vi "write TBM configuration.vi"(8 "error in":errorcluster, 10 "configuration":refnum<class "TBM configuration.lvclass">, 11 "tag bus configurable plugin editor node in":refnum<class "tag bus configurable plugin editor node.lvclass">) -> (0 "error out":errorcluster, 3 "tag bus configurable plugin editor node out":refnum<class "tag bus configurable plugin editor node.lvclass">)   [LabVIEW 2013, in "tag bus configurable plugin editor node.lvclass"]
uses:
  tag bus configurable plugin editor node.lvclass
  <vilib>/NI/Tag Bus Module Framework/root configuration/TBM configuration.lvclass
  module/configuration/tag bus configurable plugin module configuration.lvclass
  tag bus configurable plugin editor node.lvclass/tag bus configurable plugin editor node.ctl
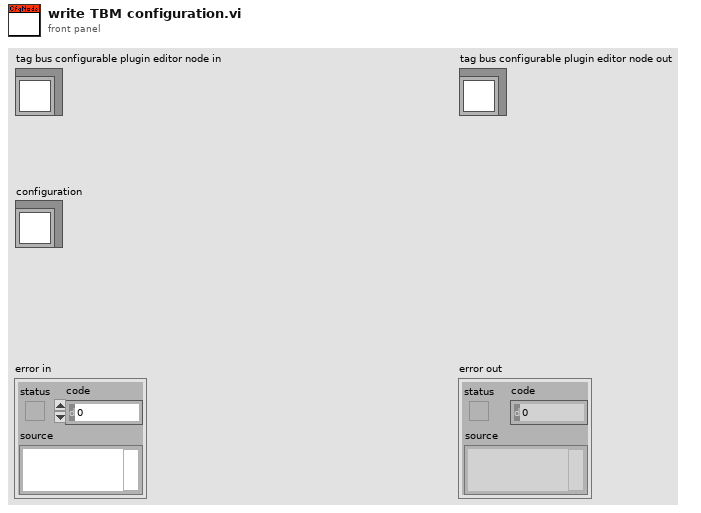
[diagram p1: front panel]
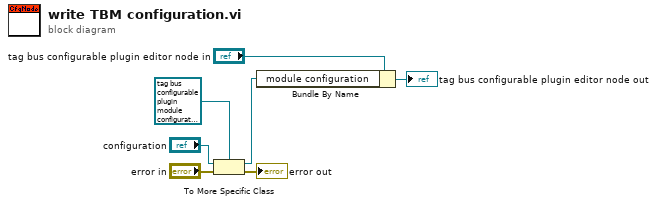
[diagram p0: block diagram]
diagram:
  n1 = To More Specific Class(target class=refnum<class "tag bus configurable plugin module configuration.lvclass"> refnum ("module configuration"), reference="configuration", error in="error in") -> (specific class reference=w1:refnum<class "tag bus configurable plugin module configuration.lvclass">, error out=→"error out":errorcluster)
  n2 = Bundle By Name(cluster="tag bus configurable plugin editor node in", "module configuration"=w1) -> (→"tag bus configurable plugin editor node out":refnum<class "tag bus configurable plugin editor node.lvclass">)
